vi "New ooWriter Report.vi"(5 "window state (normal)":T1(ring)=enum."normal", 7 "ooWriter":refnum<class "ooWriter.lvclass">, 8 "error in (no error)":errorcluster, 9 "machine name (empty)":string, 10 "template (empty)":path, 11 "display alerts? (F)":bool) -> (0 "error out":errorcluster, 3 "ooWriter out":refnum<class "ooWriter.lvclass">)   [LabVIEW 2009, in "ooWriter.lvclass"]
uses:
  ooWriter.lvclass
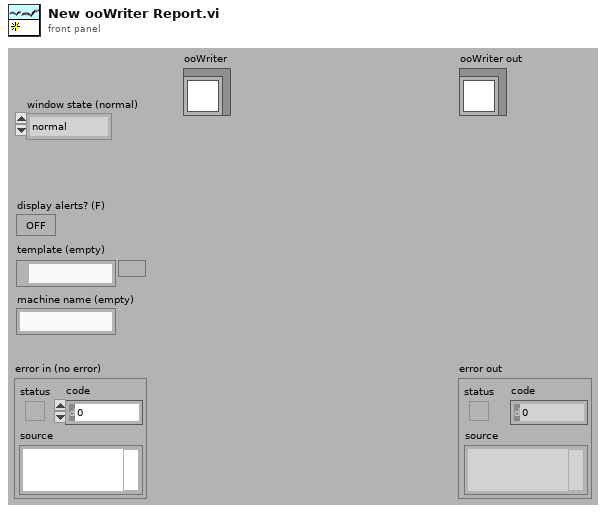
[diagram p1: front panel]
types:
  T1 = enum16{"maximized", "minimized", "normal", "no change"}
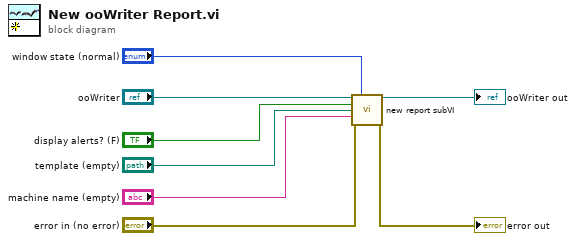
[diagram p0: block diagram]
diagram:
  n1 = call-dynamic "new report subVI.vi"("report in"="ooWriter", "window state (normal)"="window state (normal)", "display alerts? (F)"="display alerts? (F)", "template (empty)"="template (empty)", "machine name (empty)"="machine name (empty)", "error in (no error)"="error in (no error)") -> ("report out"=→"ooWriter out":refnum<class "ooWriter.lvclass">, "error out"=→"error out":errorcluster)  [unwired: 8 out]
